vi "Autonomous_Begin.vi"() -> ()   [LabVIEW 2019]
uses:
  Control 2.ctl
  <vilib>/Rock Robotics/WPI/Utilities/WPI_GetSetVariantRefNum.vi
  <vilib>/Rock Robotics/WPI/RobotDrive/WPI_RobotDriveArcadeDrive_Standard(NoSaturation).vi
  <vilib>/Rock Robotics/SystemInterfaces/DIO/FPGA_DIOPWMChannel.ctl
  <vilib>/Rock Robotics/WPI/RobotDrive/WPI_RobotDriveOpen2MotorWithVictorSPX.vi
  <vilib>/Rock Robotics/WPI/SafetyOutput/WPI_SafetyOutputConfigMenu.ctl
panel:
  in  "Turn":bool
  in  "Target Recognition":bool
  out "Next State":T1
  in  "Finish":bool
  in  "Target locked":bool
  in  "stop":bool
  in  "All balls shot":bool
  in  "Forward":bool
  in  "target recognition":bool
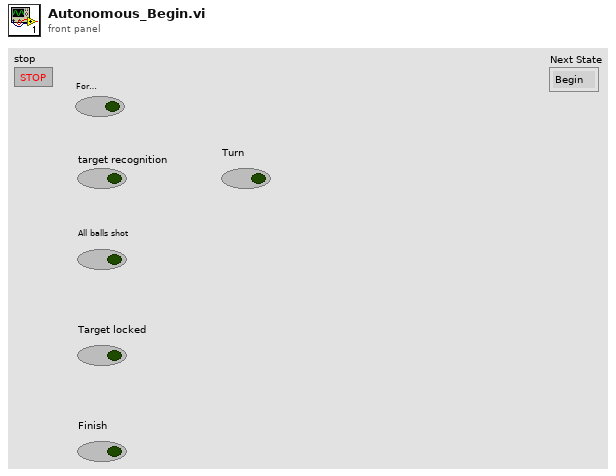
[diagram p1: front panel]
types:
  T1 = typedef "Control 2.ctl" = enum16{"Begin", "Forward", "Turn", "Aim", "Shoot", "Wait", "Finish"}
  T2 = typedef "WPI_SafetyOutputConfigMenu.ctl" = enum16{"Enable", "Disable"}
  T3 = typedef "FPGA_DIOPWMChannel.ctl" = enum8{"PWM 0", "PWM 1", "PWM 2", "PWM 3", "PWM 4", "PWM 5", "PWM 6", "PWM 7", "PWM 8", "PWM 9", "PWM MXP 0", "PWM MXP 1", "PWM MXP 2", "PWM MXP 3", "PWM MXP 4", "PWM MXP 5", "PWM MXP 6", "PWM MXP 7", "PWM MXP 8", "PWM MXP 9", "Invalid"}
  T4 = typedef "WPI_RobotDriveDevRef.ctl" = cluster{"DevStatus":errorcluster, "Motors[]":T5[], "Square Inputs":bool, "Max Output":dbl}
  T5 = typedef "WPI_MotorControlDeviceRef.ctl" = cluster{"DeviceStatus":errorcluster, "Type":T6, "PWM":cluster{"PWM Channel":T3, "DeadBand":T7}, "CAN":cluster{"Device Number":u8, "SetOutput VI Ref":variant, "GetOutput VI Ref":variant, "Enable VI Ref":variant, "Disable VI Ref":variant, "Data":variant}, "Invert":bool, "DIO PWM":cluster{"PWM \"Enable\" Channel":T3, "DIOChannel":T8, "PWM Rate":dbl}}
  T6 = typedef "WPI_MotorControlType.ctl" = enum16{"PWM", "CAN", "DIO PWM"}
  T7 = typedef "WPI_PWMDeadband.ctl" = cluster{"Name":string, "maxPositivePwm":i32, "minPositivePwm":i32, "centerPwm":i32, "maxNegativePwm":i32, "minNegativePwm":i32, "angularRange":u16}
  T8 = typedef "FPGA_DIOChannel.ctl" = enum8{"DIO 0", "DIO 1", "DIO 2", "DIO 3", "DIO 4", "DIO 5", "DIO 6", "DIO 7", "DIO 8", "DIO 9", "DIO MXP 0", "DIO MXP 1", "DIO MXP 2", "DIO MXP 3", "DIO MXP 4", "DIO MXP 5", "DIO MXP 6", "DIO MXP 7", "DIO MXP 8", "DIO MXP 9", "DIO MXP 10", "DIO MXP 11", "DIO MXP 12", "DIO MXP 13", "DIO MXP 14", "DIO MXP 15", "SPI Port CS1", "SPI Port CS2", "SPI Port CS3", "SPI Port MISO", "SPI Port MOSI", "Invalid"}
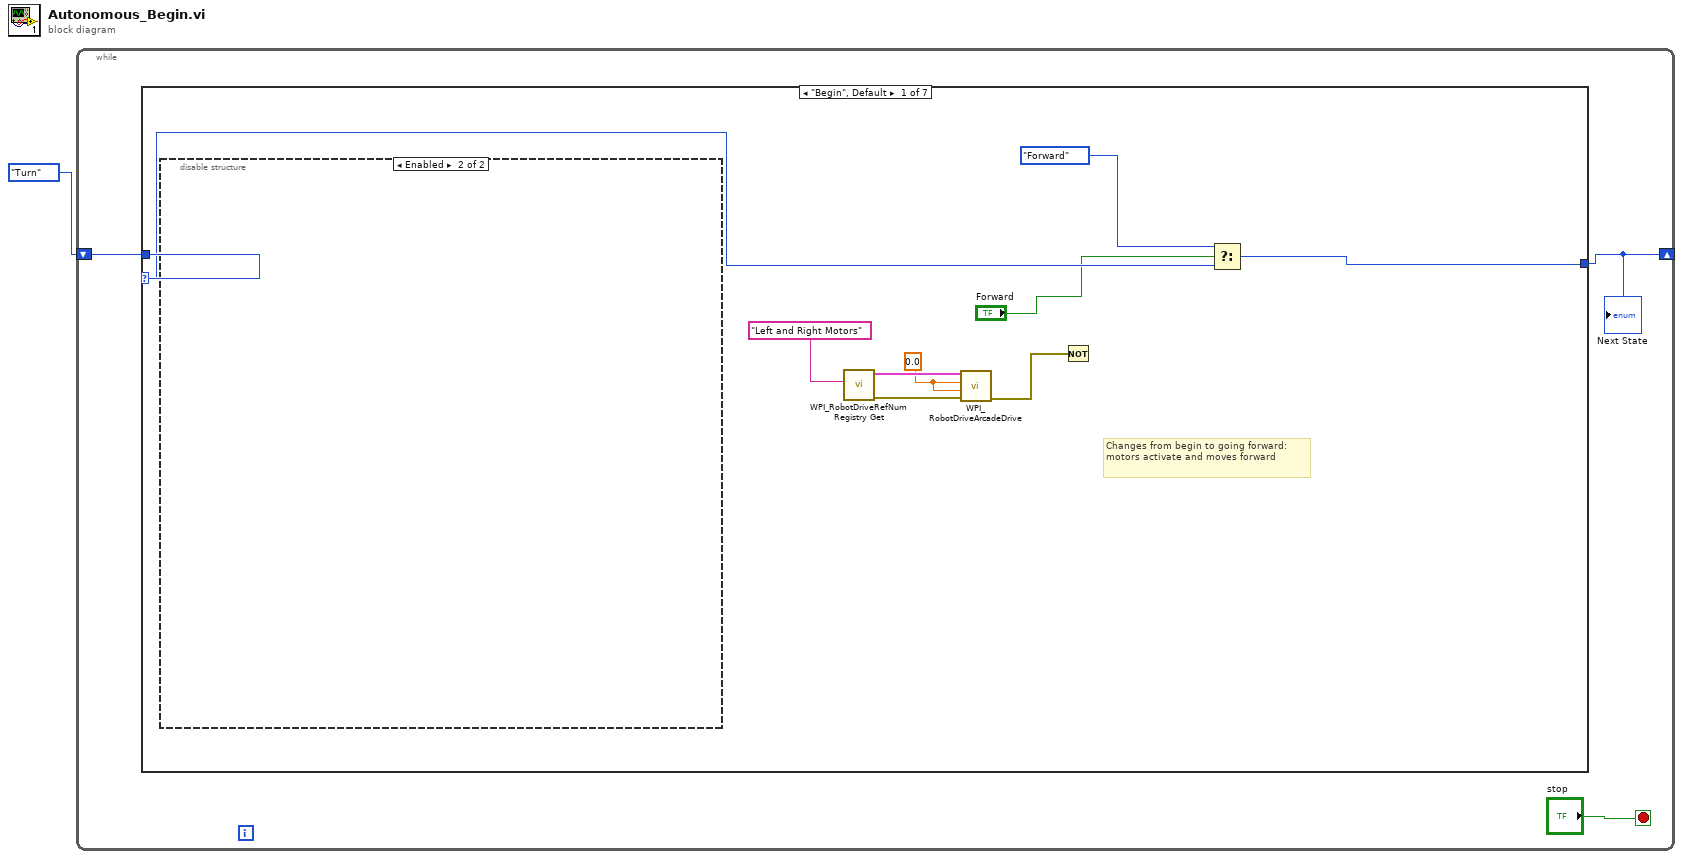
[diagram p0: block diagram]
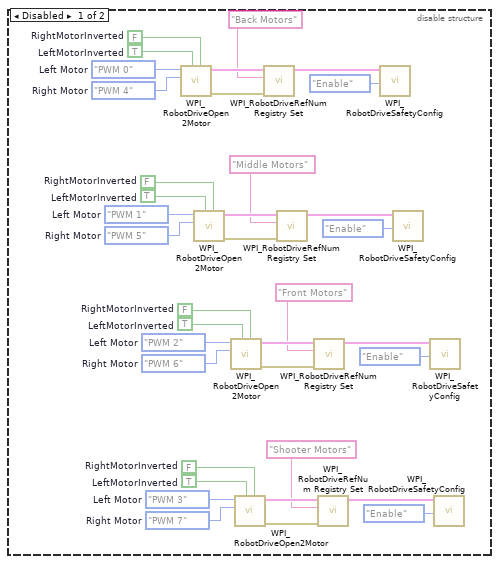
[diagram p2: hidden frame]
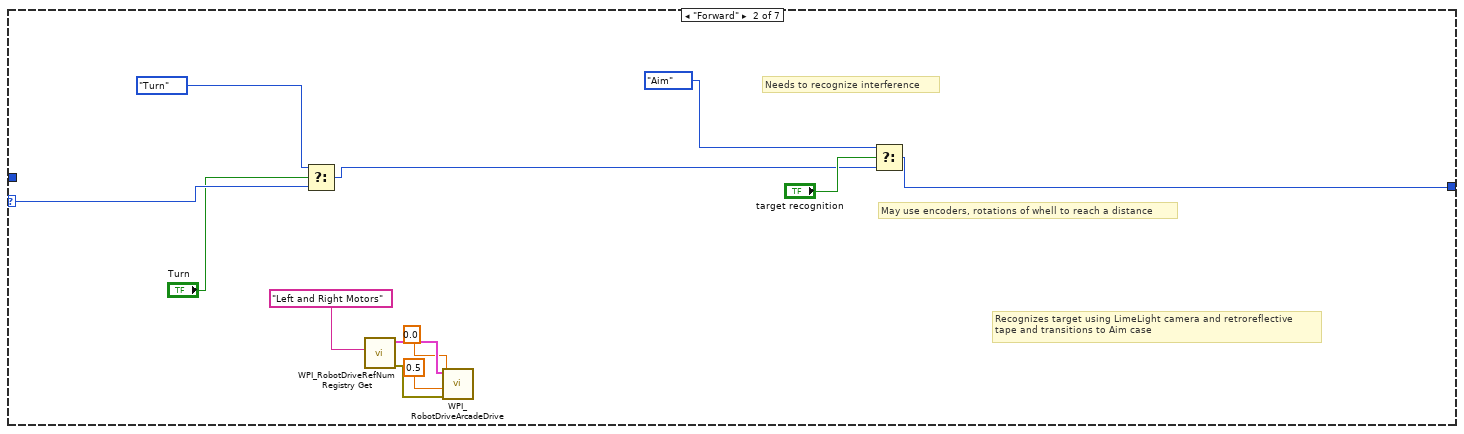
[diagram p3: hidden frame]
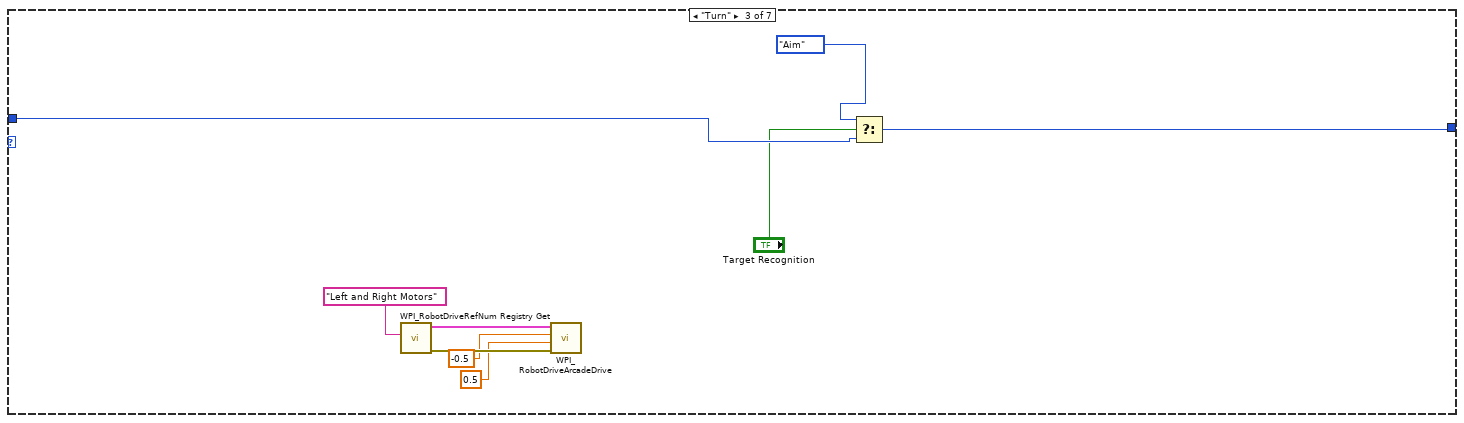
[diagram p4: hidden frame]
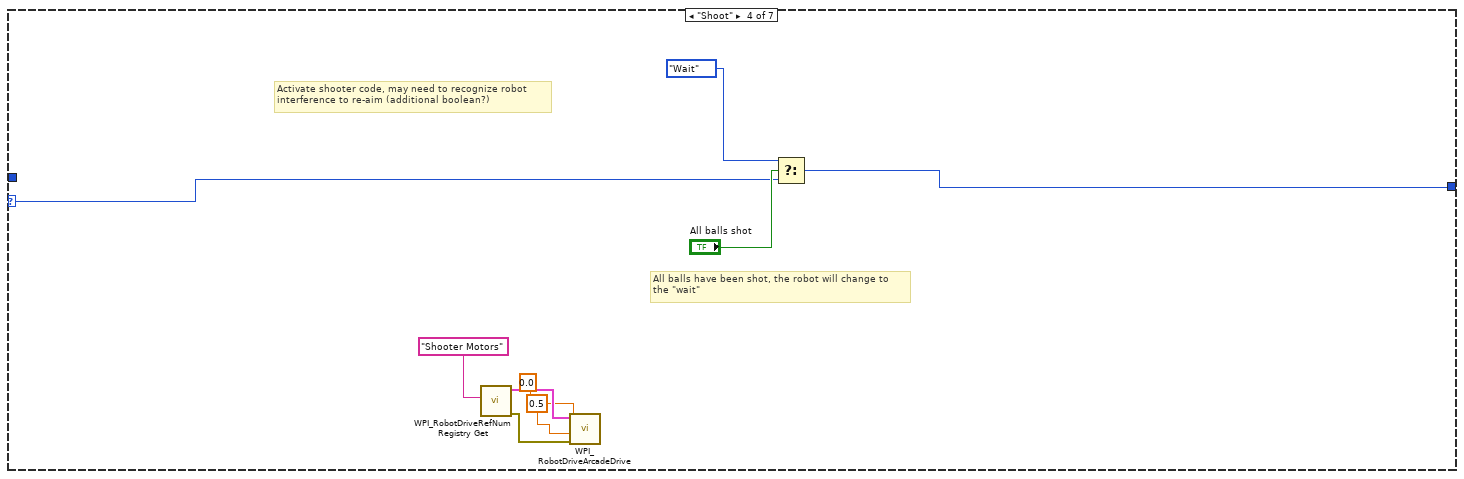
[diagram p5: hidden frame]
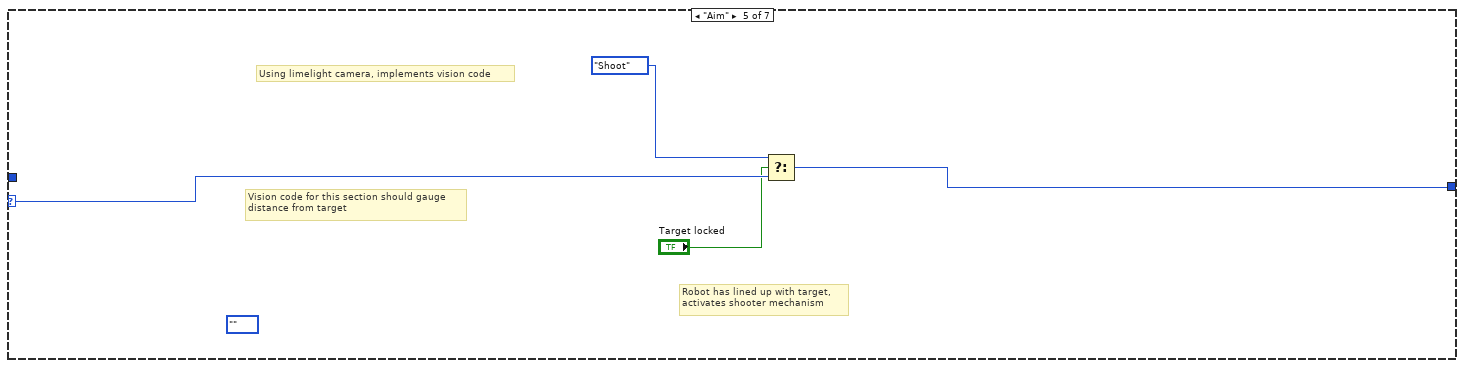
[diagram p6: hidden frame]
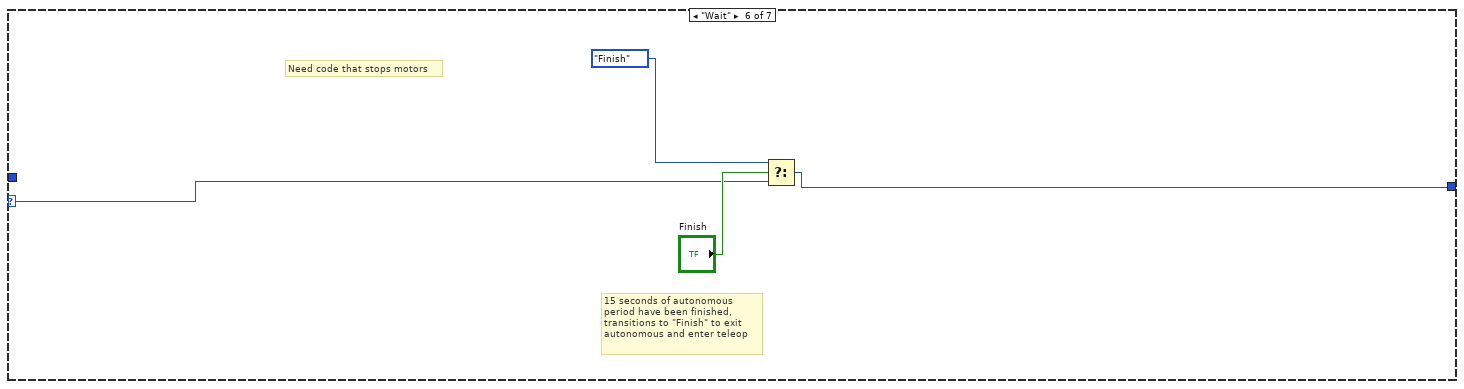
[diagram p7: hidden frame]
diagram:
  n1 = while {
    shift-right: [w3] -> _
    shift-left: Control_2."Turn" -> [w2]
    stop <- "stop" stop-if-true
    n2 = case shown="\"Begin\", Default" w2 {
      selector: w2 -> [w11 w51 _ w78 w83 w86 w88]
      tunnel: [w13 w60 w69 w77 w81 w85 w88] -> w3
      tunnel: w2 -> [_ _ w70 _ _ _ _]
      frame "Begin", Default {
        w8 = 0.0 ("X axis value")
        # "Changes from begin to going forward:\nmotors activate and moves forward"
        n3 = disable-structure shown="Enabled" {
          frame Disabled {
            w16 = FPGA_DIOPWMChannel."PWM 7"  # Right Motor
            w17 = FPGA_DIOPWMChannel."PWM 3"  # Left Motor
            w21 = TRUE  # LeftMotorInverted
            w22 = FALSE  # RightMotorInverted
            w25 = FPGA_DIOPWMChannel."PWM 6"  # Right Motor
            w26 = FPGA_DIOPWMChannel."PWM 2"  # Left Motor
            w30 = TRUE  # LeftMotorInverted
            w31 = FALSE  # RightMotorInverted
            w34 = FPGA_DIOPWMChannel."PWM 5"  # Right Motor
            w35 = FPGA_DIOPWMChannel."PWM 1"  # Left Motor
            w39 = TRUE  # LeftMotorInverted
            w40 = FALSE  # RightMotorInverted
            w43 = FPGA_DIOPWMChannel."PWM 4"  # Right Motor
            w44 = FPGA_DIOPWMChannel."PWM 0"  # Left Motor
            w48 = TRUE  # LeftMotorInverted
            w49 = FALSE  # RightMotorInverted
            n4 = call-poly <vilib>:"WPI_RobotDriveOpen2Motor.vi"("Right Motor Inverted"=w49, "Left Motor Inverted"=w48, "Right Motor"=w43, "Left Motor"=w44) -> ("error out"=w45:errorcluster, "RobotDriveDevRef"=w47:T4)  [unwired: 1 in, 5 out]
            n5 = call-poly <vilib>:"WPI_RobotDriveOpen2Motor.vi"("Right Motor Inverted"=w40, "Left Motor Inverted"=w39, "Right Motor"=w34, "Left Motor"=w35) -> ("error out"=w36:errorcluster, "RobotDriveDevRef"=w38:T4)  [unwired: 1 in, 5 out]
            n6 = call-poly <vilib>:"WPI_RobotDriveOpen2Motor.vi"("Right Motor Inverted"=w31, "Left Motor Inverted"=w30, "Right Motor"=w25, "Left Motor"=w26) -> ("error out"=w27:errorcluster, "RobotDriveDevRef"=w29:T4)  [unwired: 1 in, 5 out]
            n7 = call-poly <vilib>:"WPI_RobotDriveOpen2Motor.vi"("Right Motor Inverted"=w22, "Left Motor Inverted"=w21, "Right Motor"=w16, "Left Motor"=w17) -> ("error out"=w18:errorcluster, "RobotDriveDevRef"=w20:T4)  [unwired: 1 in, 5 out]
            n8 = call <vilib>:"WPI_RobotDriveRefNum Registry Set.vi"("error in (no error)"=w45, "refnum name"="Back Motors", "RobotDriveDevRef"=w47) -> ("RobotDriveDevRef"=w42:T4)  [unwired: 1 in, 7 out]
            n9 = call <vilib>:"WPI_RobotDriveRefNum Registry Set.vi"("error in (no error)"=w36, "refnum name"="Middle Motors", "RobotDriveDevRef"=w38) -> ("RobotDriveDevRef"=w33:T4)  [unwired: 1 in, 7 out]
            n10 = call <vilib>:"WPI_RobotDriveRefNum Registry Set.vi"("error in (no error)"=w27, "refnum name"="Front Motors", "RobotDriveDevRef"=w29) -> ("RobotDriveDevRef"=w24:T4)  [unwired: 1 in, 7 out]
            n11 = call <vilib>:"WPI_RobotDriveRefNum Registry Set.vi"("error in (no error)"=w18, "refnum name"="Shooter Motors", "RobotDriveDevRef"=w20) -> ("RobotDriveDevRef"=w15:T4)  [unwired: 1 in, 7 out]
            n12 = call <vilib>:"WPI_RobotDriveSafetyConfig.vi"("mode"=WPI_SafetyOutputConfigMenu."Enable", "RobotDriveDevRef"=w42) -> ()  [unwired: 8 in, 2 out]
            n13 = call <vilib>:"WPI_RobotDriveSafetyConfig.vi"("mode"=WPI_SafetyOutputConfigMenu."Enable", "RobotDriveDevRef"=w33) -> ()  [unwired: 8 in, 2 out]
            n14 = call <vilib>:"WPI_RobotDriveSafetyConfig.vi"("mode"=WPI_SafetyOutputConfigMenu."Enable", "RobotDriveDevRef"=w24) -> ()  [unwired: 8 in, 2 out]
            n15 = call <vilib>:"WPI_RobotDriveSafetyConfig.vi"("mode"=WPI_SafetyOutputConfigMenu."Enable", "RobotDriveDevRef"=w15) -> ()  [unwired: 8 in, 2 out]
          }
          frame Enabled {
          }
        }
        n16 = call <vilib>:"WPI_RobotDriveRefNum Registry Get.vi"("refnum name"="Left and Right Motors") -> ("error out"=w7:errorcluster, "RobotDriveDevRef"=w9:T4)  [unwired: 1 in, 8 out]
        n17 = call-poly <vilib>:"WPI_RobotDriveArcadeDrive.vi"("error in (no error)"=w7, "Y axis value"=w8, "X axis value"=w8, "RobotDriveDevRef"=w9) -> ("error out"=w6:errorcluster)  [unwired: 5 in, 2 out]
        n18 = Not(x=w6) -> ()  [unwired: 1 out]
        n19 = Select(t=Control_2."Forward", s="Forward", f=w11) -> (s? t:f=w13:T1)
      }
      frame "Forward" {
        # "May use encoders, rotations of whell to reach a distance"
        # "Needs to recognize interference"
        # "Recognizes target using LimeLight camera and retroreflective \ntape and transitions to Aim case"
        n20 = Select(t=Control_2."Turn", s="Turn", f=w51) -> (s? t:f=w52:T1)
        n21 = call <vilib>:"WPI_RobotDriveRefNum Registry Get.vi"("refnum name"="Left and Right Motors") -> ("error out"=w56:errorcluster, "RobotDriveDevRef"=w57:T4)  [unwired: 1 in, 8 out]
        n22 = call-poly <vilib>:"WPI_RobotDriveArcadeDrive.vi"("error in (no error)"=w56, "Y axis value"=0.5, "X axis value"=0.0, "RobotDriveDevRef"=w57) -> ()  [unwired: 5 in, 3 out]
        n23 = Select(t=Control_2."Aim", s="target recognition", f=w52) -> (s? t:f=w60:T1)
      }
      frame "Turn" {
        n24 = call <vilib>:"WPI_RobotDriveRefNum Registry Get.vi"("refnum name"="Left and Right Motors") -> ("error out"=w66:errorcluster, "RobotDriveDevRef"=w65:T4)  [unwired: 1 in, 8 out]
        n25 = call-poly <vilib>:"WPI_RobotDriveArcadeDrive.vi"("error in (no error)"=w66, "Y axis value"=0.5, "X axis value"=-0.5, "RobotDriveDevRef"=w65) -> ()  [unwired: 5 in, 3 out]
        n26 = Select(t=Control_2."Aim", s="Target Recognition", f=w70) -> (s? t:f=w69:T1)
      }
      frame "Shoot" {
        # "Activate shooter code, may need to recognize robot\ninterference to re-aim (additional boolean?)"
        # "All balls have been shot, the robot will change to\nthe \"wait\""
        n27 = call <vilib>:"WPI_RobotDriveRefNum Registry Get.vi"("refnum name"="Shooter Motors") -> ("error out"=w73:errorcluster, "RobotDriveDevRef"=w74:T4)  [unwired: 1 in, 8 out]
        n28 = call-poly <vilib>:"WPI_RobotDriveArcadeDrive.vi"("error in (no error)"=w73, "Y axis value"=0.5, "X axis value"=0.0, "RobotDriveDevRef"=w74) -> ()  [unwired: 5 in, 3 out]
        n29 = Select(t=Control_2."Wait", s="All balls shot", f=w78) -> (s? t:f=w77:T1)
      }
      frame "Aim" {
        (unwired) enum16{""}.""
        # "Vision code for this section should gauge\ndistance from target"
        # "Using limelight camera, implements vision code"
        # "Robot has lined up with target, \nactivates shooter mechanism"
        n30 = Select(t=Control_2."Shoot", s="Target locked", f=w83) -> (s? t:f=w81:T1)
      }
      frame "Wait" {
        # "Need code that stops motors"
        # "15 seconds of autonomous\nperiod have been finished, \ntransitions to \"Finish\" to exit \nautonomous and enter teleop"
        n31 = Select(t=Control_2."Finish", s="Finish", f=w86) -> (s? t:f=w85:T1)
      }
      frame "Finish" {
        # "Links code to teleop"
      }
    }
    "Next State" <- w3
  }
